vi "Bertta_v09_6.vi"() -> ()   [LabVIEW 2015]
uses:
  x64/Debug/BERTTA.dll
panel:
  out "TIME array":dbl[](array[numeric])
  out "TEMP array":dbl[](array[numeric])
  out "element":bool
  out "Started:":string
  in  "SHUTDOWN":bool
  in  "MASTER CONTROL":bool
  in  "Tab Control":T1(tab)
  in  "Read Seq":bool
  in  "Save Seq":bool
  in  "Configuration file":path=path "C:/Users/shresplab/Desktop/BerttaConfiguration.lvm" caption="Filename"
  in  "OK Button 2":bool
  out "Boolean":bool
  in  "User (initials)":string
  in  "Project name":string
  in  "Description":string
  out "Output file":string
  out "PUMP 3":bool
  out "Target amount":dbl
  out "Scale weight":dbl
  out "Amount now":dbl
  out "Flow rate":dbl
  out "Time to target":dbl format="%<%H:%M:%S>t"
  out "Current step":dbl
  out "Target amount":dbl
  out "Amount now":dbl
  out "Amount now":dbl
  out "Target amount":dbl
  out "Current step":dbl
  out "Time to target":dbl format="%<%H:%M:%S>t"
  out "Flow rate":dbl
  out "Amount now":dbl
  out "Scale weight":dbl
  out "Target amount":dbl
  out "PUMP 2":bool
  out "Sensor OK 6":bool
  out "Sensor OK 5":bool
  out "Sensor OK 4":bool
  out "Sensor OK 3":bool
  in  "OK Button":bool
  in  "Add comment":string
  out "PUMP 1":bool
  out "Target amount":dbl
  out "Scale weight":dbl
  out "Amount now":dbl
  out "Flow rate":dbl
  out "Time to target":dbl format="%<%H:%M:%S>t"
  out "Current step":dbl
  out "Target amount":dbl
  out "Amount now":dbl
  out "Tr":dbl
  out "Tj in":dbl
  out "Tj out":dbl
  out "T set":dbl
  out "Current step":i32
  out "RPM":dbl
  out "Torque 2":dbl
  out "Waveform Chart 5":dynamicdata(graph)
  out "Waveform Chart 6":dynamicdata(graph)
  out "Waveform Chart 7":dynamicdata(graph)
  in  "Tab Control 2":T2(tab)
  out "Waveform Chart 3":dynamicdata(graph)
  out "Waveform Chart 8":dynamicdata(graph)
  out "Waveform Chart 11":dynamicdata(graph)
  out "Waveform Chart 13":dynamicdata(graph)
  out "Waveform Chart 9":dynamicdata(graph)
  out "Table":string[][](table)=[["14.8.2017 18.06.59", "0,000000", "417,670000", "-0,150000", "1,000000", "22,220000", "23,366837", "23,574959", "23,985852", "23,690000", "240,000000", "4,000000", "0,000000", "397,000000", "-397,000000", "1,000000"], ["14.8.2017 18.07.06", "0,000000", "417,640000", "-0,120000", "1,000000", "22,220000", "23,763115", "23,906257", "23,985694", "23,680000", "240,000000", "4,000000", "0,000000", "397,000000", "-397,000000", "1,000000"], ["14.8.2017 18.07.13", "0,000000", "417,640000", "-0,120000", "1,000000", "22,220000", "23,965922", "24,013440", "23,984906", "23,670000", "240,000000", "4,100000", "3,000000", "397,000000", "-397,000000", "1,000000"], ["14.8.2017 18.07.21", "0,000000", "417,640000", "-0,120000", "1,000000", "22,220000", "23,943860", "23,900110", "23,987113", "23,670000", "240,000000", "4,000000", "0,000000", "397,000000", "-397,000000", "1,000000"], ["14.8.2017 18.07.28", "0,000000", "417,640000", "-0,120000", "1,000000", "22,220000", "23,736328", "23,600018", "23,989004", "23,660000", "240,000000", "4,000000", "0,000000", "397,000000", "-397,000000", "1,000000"], ["14.8.2017 18.07.36", "0,000000", "417,640000", "-0,120000", "1,000000", "22,220000", "23,480910", "23,324538", "23,991053", "23,660000", "240,000000", "4,000000", "0,000000", "397,000000", "-397,000000", "1,000000"], ["14.8.2017 18.07.43", "0,000000", "417,640000", "-0,120000", "2,000000", "22,220000", "23,195579", "23,008270", "23,999093", "23,650000", "240,000000", "4,000000", "0,000000", "397,000000", "-397,000000", "1,000000"], ["14.8.2017 18.07.51", "0,000000", "417,650000", "-417,650000", "1,000000", "22,220000", "22,862541", "22,649021", "24,003979", "23,650000", "240,000000", "4,000000", "0,000000", "397,000000", "-397,000000", "2,000000"], ["14.8.2017 18.07.58", "0,000000", "417,640000", "0,010000", "1,000000", "22,220000", "22,541353", "22,354878", "24,005398", "23,650000", "240,000000", "4,000000", "0,000000", "397,000000", "-397,000000", "1,000000"], ["14.8.2017 18.08.06", "0,000000", "417,640000", "0,010000", "1,000000", "22,220000", "22,347931", "22,253738", "24,007605", "23,640000", "240,000000", "4,100000", "0,000000", "397,000000", "-397,000000", "1,000000"], ["14.8.2017 18.08.13", "0,000000", "417,640000", "0,010000", "1,000000", "22,220000", "22,329030", "22,302102", "24,006028", "23,640000", "240,000000", "4,000000", "0,000000", "395,820000", "-395,820000", "1,000000"], ["14.8.2017 18.08.20", "0,000000", "417,640000", "0,010000", "1,000000", "22,220000", "22,466849", "22,511320", "24,002403", "23,630000", "240,000000", "4,000000", "0,000000", "395,830000", "-0,010000", "1,000000"], ["14.8.2017 18.08.28", "0,000000", "417,640000", "0,010000", "1,000000", "22,220000", "22,707062", "22,835101", "24,000984", "23,620000", "240,000000", "4,000000", "0,000000", "395,830000", "-0,010000", "1,000000"], ["14.8.2017 18.08.35", "0,000000", "417,640000", "0,010000", "1,000000", "22,220000", "23,054104", "23,232979", "24,001299", "23,600000", "240,000000", "4,000000", "0,000000", "395,830000", "-0,010000", "1,000000"], ["14.8.2017 18.08.43", "0,000000", "417,640000", "0,010000", "1,000000", "22,220000", "23,412371", "23,522793", "24,002560", "23,590000", "240,000000", "4,000000", "0,000000", "395,820000", "0,000000", "1,000000"], ["14.8.2017 18.08.51", "0,000000", "417,640000", "0,010000", "1,000000", "22,220000", "23,596247", "23,656125", "24,003821", "23,580000", "240,000000", "4,000000", "0,000000", "395,820000", "0,000000", "1,000000"]]
  in  "Reset":bool
  in  "Numeric 4":dbl=20.0
  in  "Numeric 3":dbl=30.0
  in  "Numeric 2":dbl=40.0
  in  "Numeric 1":dbl=30.0
  in  "Numeric":dbl=20.0
  out "Boolean 12":bool
  out "Boolean 7":bool
  out "Boolean 6":bool
  out "Boolean 5":bool
  out "Boolean 4":bool
  out "Boolean 19":bool
  in  "Numeric 5":dbl=5.0
  in  "Numeric 6":dbl=5.0
  in  "Numeric 7":dbl=5.0
  in  "Numeric 8":dbl=5.0
  in  "T ext / T ext 2":enum32{"External 1", "External 2"}(radio)
  out "Sensor OK":bool
  in  "T fail":dbl=20.0
  in  "?":bool
  in  "T manual setpoint":dbl=20.0
  in  "Lauda port":dbl=9.0
  in  "Manual select":enum32{"Tr", "Tj"}(radio)
  in  "PAUSE":bool
  out "Waveform Chart":dynamicdata(graph)
  out "T external 2":dbl
  out "result":bool
  out "Led11 5":bool
  in  "Port":i32=10
  in  "Radio Buttons 4":enum32{"Reglo Digital", "Reglo Analog", "PAM"}(radio)
  out "Speed":dbl
  out "mA":dbl format="%#_2g"
  in  "Port":i32=16
  out "RPM":dbl format="%_4f"
  out "Led10 3":bool
  out "Led9 3":bool
  out "Led8 3":bool
  out "Led7 3":bool
  out "Led6 3":bool
  out "Led5 3":bool
  out "Led4 3":bool
  out "Led3 3":bool
  out "Led2 3":bool
  out "Led1 3":bool
  in  "PumpSeq 4":dbl[][](array[numeric])=[[1.0, 1.0, 7.0], [2.0, 1.0, 2.0], [3.0, 1.0, 100.0], [0.0, 0.0, 0.0], [0.0, 0.0, 0.0], [0.0, 0.0, 0.0], [0.0, 0.0, 0.0], [0.0, 0.0, 0.0], [0.0, 0.0, 0.0], [0.0, 0.0, 0.0], [0.0, 1.0, 0.0]]
  in  "?":bool
  out "Flow rate (g/min)":dbl
  out "Scale reading":dbl
  out "Step amount now":dbl
  in  "Grams / min":dbl
  out "Waveform Chart 14":dynamicdata(graph)
  in  "?":bool
  out "Total amount now":dbl
  out "Total time 4":dbl
  out "Total amount target 4":dbl
  out "Led11 4":bool
  in  "Reset 5":bool
  out "elapsed / step":i32
  out "Time to target":dbl format="%<%H:%M:%S>t"
  out "Led11":bool
  in  "Port":i32=11
  in  "Radio Buttons 2":enum32{"Reglo Digital", "Reglo Analog", "PAM"}(radio)
  out "Speed":dbl
  out "mA":dbl format="%#_2g"
  in  "Port":i32=15
  out "RPM":dbl format="%_4f"
  out "Led10":bool
  out "Led9":bool
  out "Led8":bool
  out "Led7":bool
  out "Led6":bool
  out "Led5":bool
  out "Led4":bool
  out "Led3":bool
  out "Led2":bool
  out "Led1":bool
  in  "PumpSeq 2":dbl[][](array[numeric])=[[1.0, 1.0, 7.0], [2.0, 1.0, 2.0], [3.0, 1.0, 100.0], [0.0, 0.0, 0.0], [0.0, 0.0, 0.0], [0.0, 0.0, 0.0], [0.0, 0.0, 0.0], [0.0, 0.0, 0.0], [0.0, 0.0, 0.0], [0.0, 0.0, 0.0], [0.0, 1.0, 0.0]]
  in  "?":bool
  out "Flow rate (g/min)":dbl
  out "Scale reading":dbl
  out "Step amount now":dbl
  in  "Grams / min":dbl
  out "Waveform Chart 10":dynamicdata(graph)
  in  "?":bool
  out "Total amount now":dbl
  out "Total time 2":dbl
  out "Total amount target 2":dbl
  out "Led11":bool
  in  "Reset 3":bool
  out "elapsed / step":i32
  out "Time to target":dbl format="%<%H:%M:%S>t"
  out "Led11 3":bool
  in  "Port":i32=12
  in  "Radio Buttons 3":enum32{"Reglo Digital", "Reglo Analog", "PAM"}(radio)
  out "Speed":dbl
  out "mA":dbl format="%#_2g"
  in  "Port":i32=14
  out "RPM":dbl format="%_4f"
  out "Led10 2":bool
  out "Led9 2":bool
  out "Led8 2":bool
  out "Led7 2":bool
  out "Led6 2":bool
  out "Led5 2":bool
  out "Led4 2":bool
  out "Led3 2":bool
  out "Led2 2":bool
  out "Led1 2":bool
  in  "PumpSeq 3":dbl[][](array[numeric])=[[1.0, 1.0, 7.0], [2.0, 1.0, 2.0], [3.0, 1.0, 100.0], [0.0, 0.0, 0.0], [0.0, 0.0, 0.0], [0.0, 0.0, 0.0], [0.0, 0.0, 0.0], [0.0, 0.0, 0.0], [0.0, 0.0, 0.0], [0.0, 0.0, 0.0], [0.0, 1.0, 0.0]]
  in  "?":bool
  out "Flow rate (g/min)":dbl
  out "Scale reading":dbl
  out "Step amount now":dbl
  in  "Grams / min":dbl
  out "Waveform Chart 12":dynamicdata(graph)
  in  "?":bool
  out "Total amount now":dbl
  out "Total time 3":dbl
  out "Total amount target 3":dbl
  out "Led11 2":bool
  in  "Reset 4":bool
  out "elapsed / step":i32
  out "Time to target":dbl format="%<%H:%M:%S>t"
  in  "Bypass select 2":enum32{"Remote", "Manual"}(radio)=enum."Manual"
  in  "Port":dbl=13.0
  out "RPM":dbl
  out "Torque":dbl
  in  "Set RPM":dbl(slide) scale=0.0..2000.0
  out "Waveform Chart 4":dynamicdata(graph)
  out "DAQ 9217 (PT100)":errorcluster
  # "Temperature sensor:"
  # "Manual control:"
  # "PUMP & SCALE 1"
  # "STEP"
  # "TOTAL"
  # "PUMP & SCALE 2"
  # "STEP"
  # "TOTAL"
  # "PUMP & SCALE 3"
  # "STEP"
  # "TOTAL"
  # "Manual control"
  # "Secondary temperature sensor"
  # "Device communication"
  # "Temp"
  # "Time"
  # "Grams    /   min"
  # "End of sequence"
  # "Manual control"
  # "Device communication"
  # "Pump configuration"
  # "Scale configuration"
  # "SCALE 1"
  # "Grams    /   min"
  # "End of sequence"
  # "Manual control"
  # "Device communication"
  # "Pump configuration"
  # "Scale configuration"
  # "SCALE 2"
  # "Grams    /   min"
  # "End of sequence"
  # "Manual control"
  # "Device communication"
  # "Pump configuration"
  # "Scale configuration"
  # "SCALE 3"
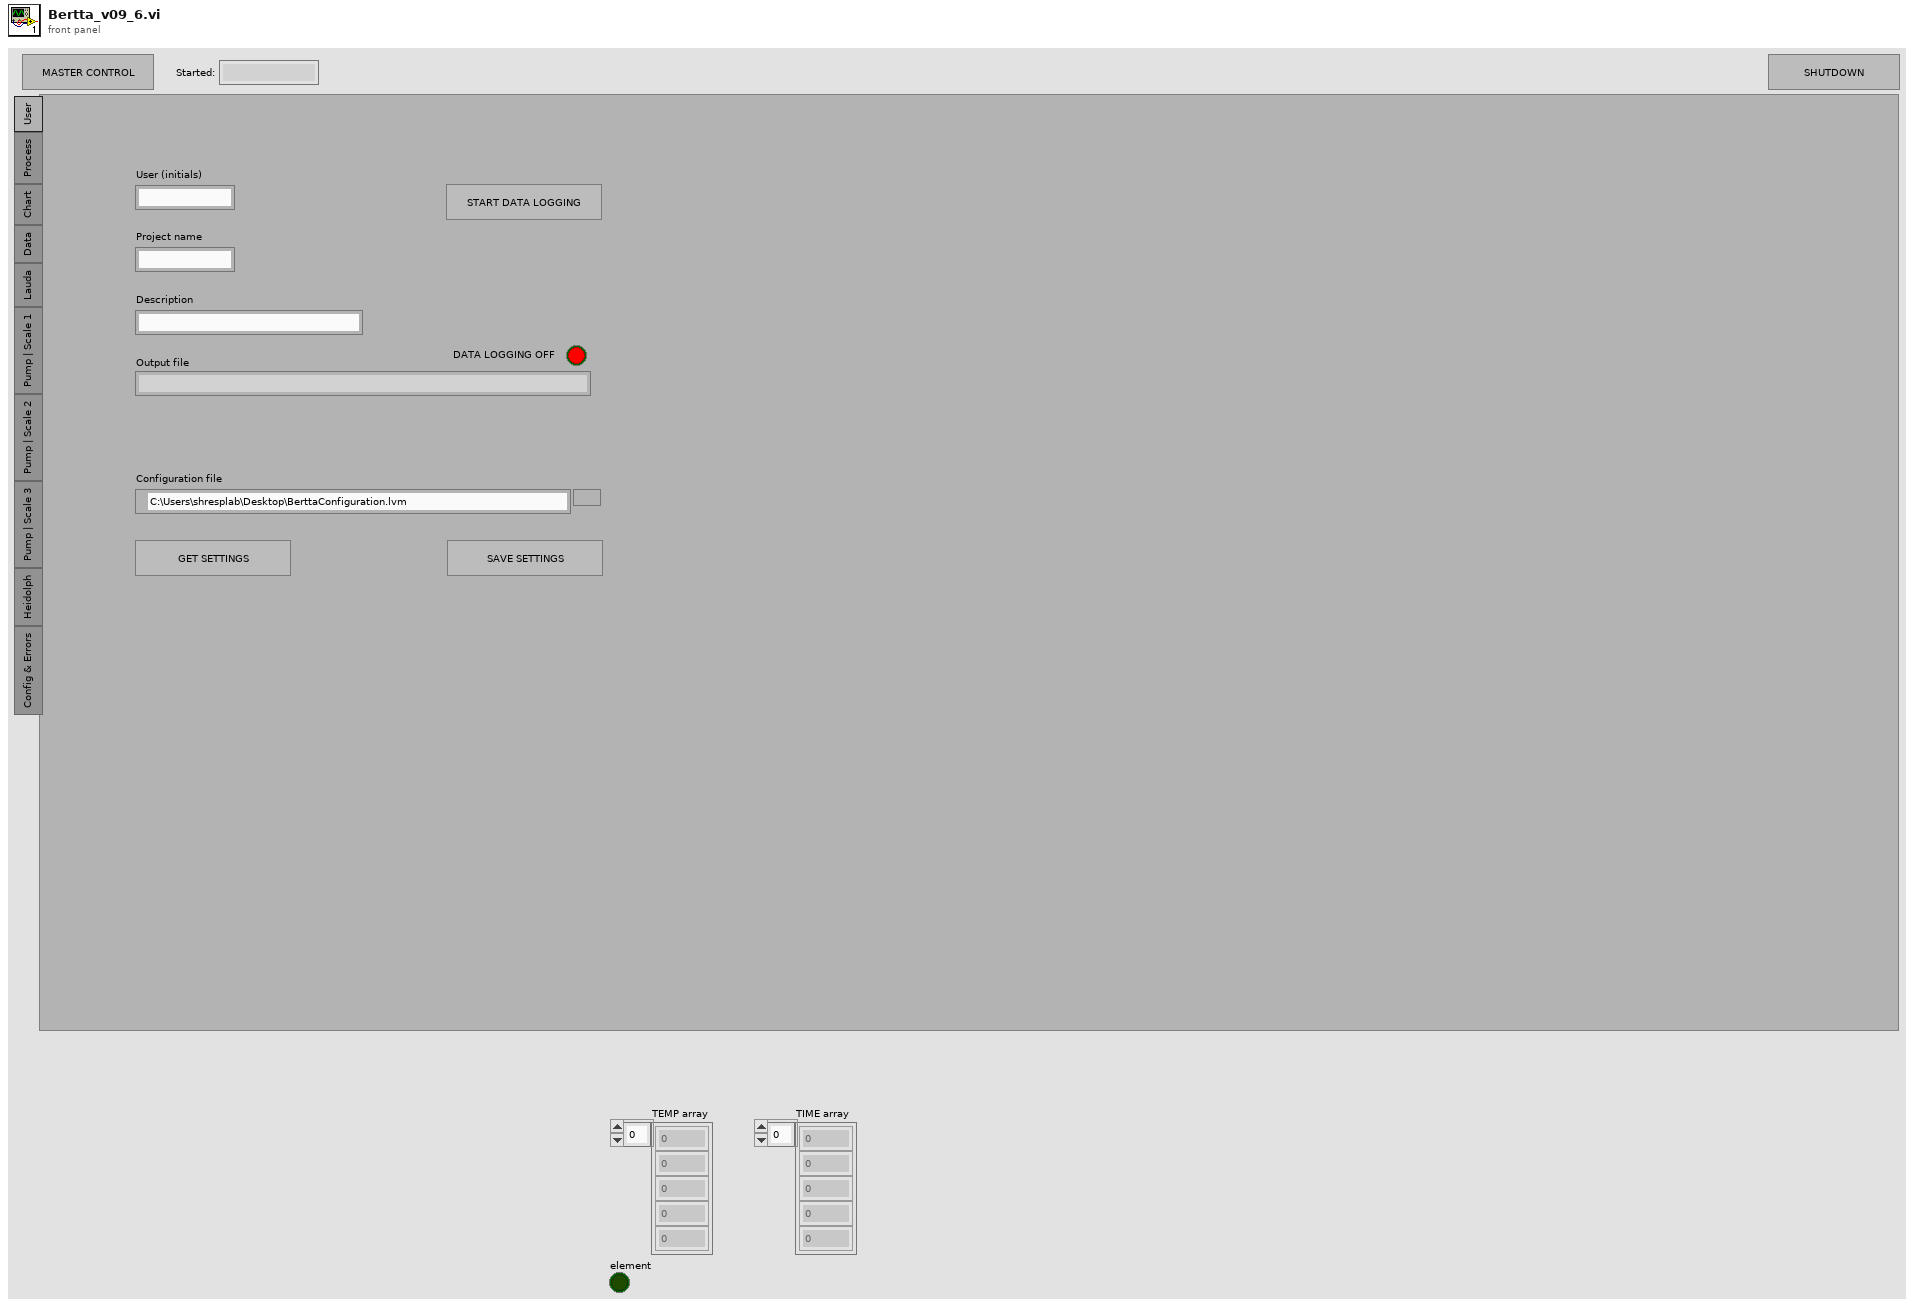
[diagram p1: front panel]
types:
  T1 = enum32{"User", "Process", "Chart", "Data", "Lauda", "Pump | Scale 1", "Pump | Scale 2", "Pump | Scale 3", "Heidolph", "Config & Errors"}
  T2 = enum32{"Temperatures", "Scale / Pump 1", "Scale / Pump 2", "Scale / Pump 3", "RPM / torque"}
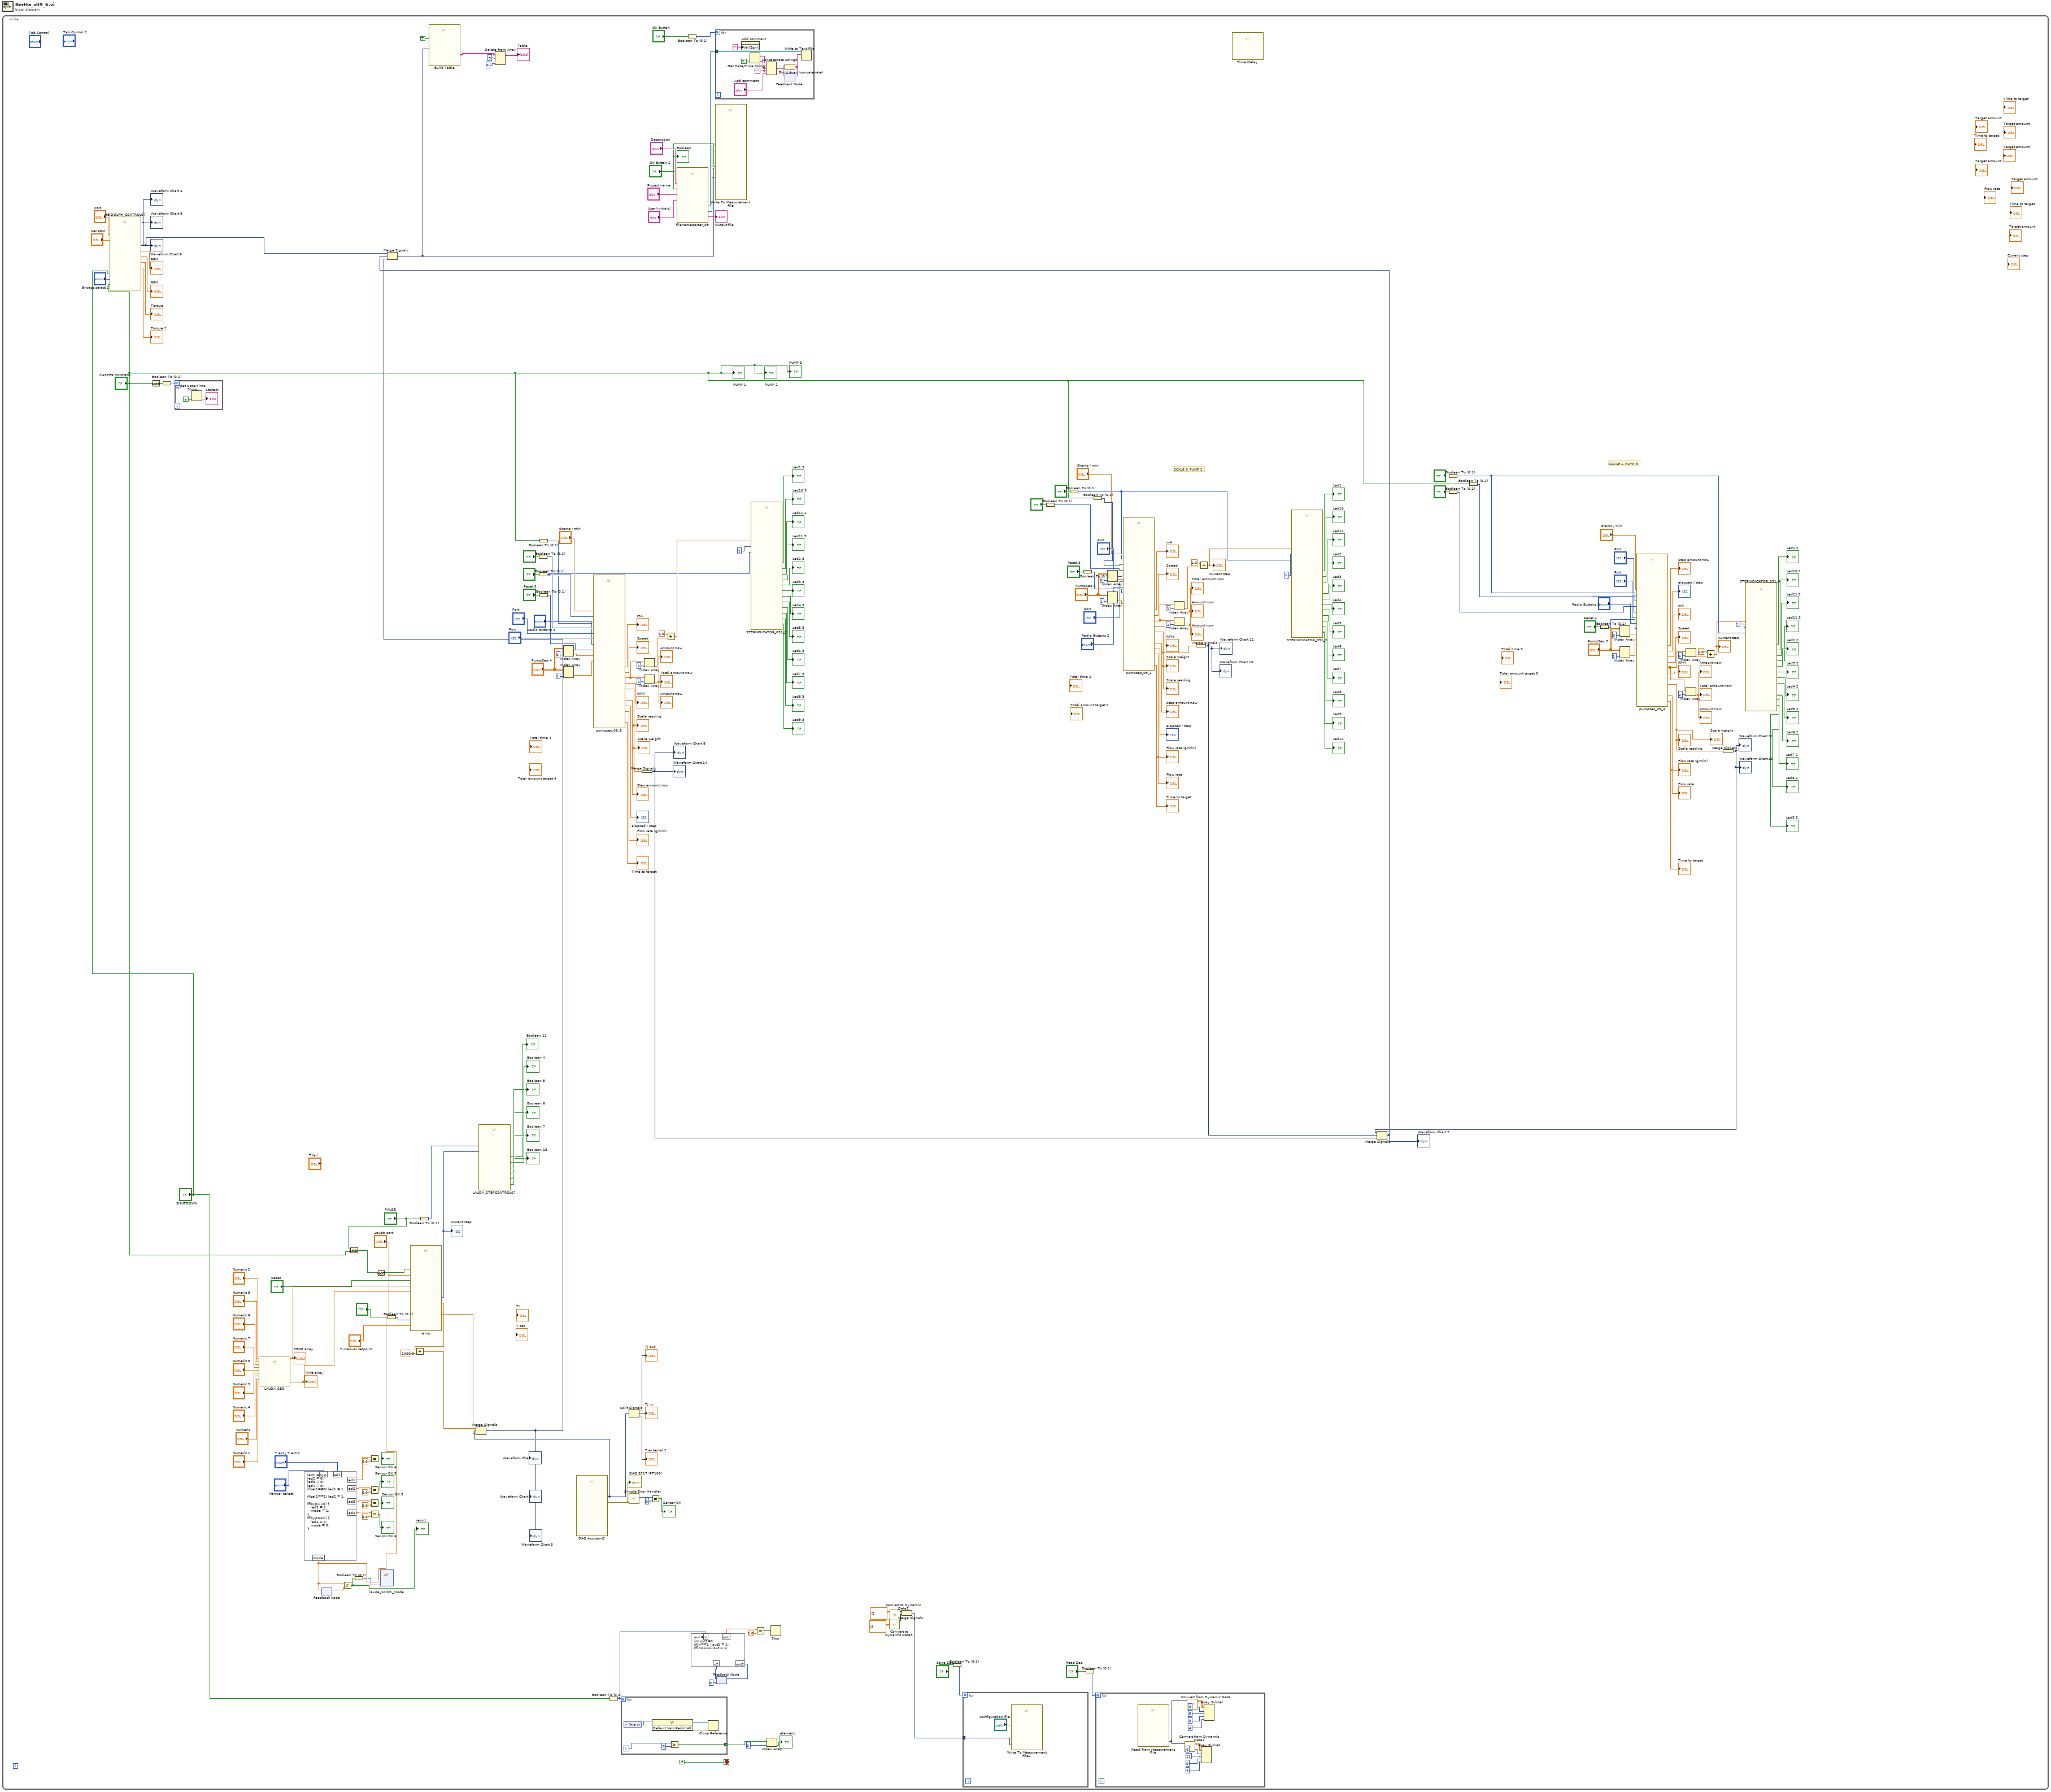
[diagram p0: block diagram]
diagram:
  n1 = while {
    stop <- FALSE stop-if-true
    # "SCALE & PUMP 3"
    # "SCALE & PUMP 2"
    n2 = call "HEIDOLPH_CONTROL07.vi"("master"="MASTER CONTROL", "shutdown"="SHUTDOWN", "Bypass select"="Bypass select 2", "Set RPM"="Set RPM", "Device port"="Port") -> ("Dynamic Data"=w235:dynamicdata, "RPM"=→"RPM":dbl, "RPM 2"=→"RPM":dbl, "Torque"=→"Torque":dbl, "Torque 2"=→"Torque 2":dbl)  [unwired: 2 in]
    "Waveform Chart 4" <- w235
    "Waveform Chart 6" <- w235
    "Waveform Chart 9" <- w235
    n3 = Not(x="MASTER CONTROL") -> (.not. x?=w220:bool)
    n4 = Boolean To (0,1)(Boolean=w220) -> (0, 1=w221:i16)
    n5 = for {
      N: w221 -> [_]
      n6 = Get Date/Time String(want seconds? (F)=TRUE) -> (time string=→"Started:":string)  [unwired: 2 in, 1 out]
    }
    n7 = call "LAUDA_SEQ.vi"("Numeric 2"="Numeric 2", "Numeric 1"="Numeric 1", "Numeric"="Numeric", "Numeric 5"="Numeric 5", "Numeric 6"="Numeric 6", "Numeric 7"="Numeric 7", "Numeric 8"="Numeric 8", "Numeric 3"="Numeric 3", "Numeric 4"="Numeric 4") -> ("output array"=w113:dbl[], "output array 2"=w112:dbl[])  [unwired: 5 in]
    "TEMP array" <- w113
    "TIME array" <- w112
    n8 = formula code="led1 = 0;\nled2 = 0;\nled3 = 0;\nled4 = 0;\nif(sel1==0) led1 = 1;\n\nif(sel1==1) led2 = 1;\n\nif(byp==0) {\n   led3 = 1;\n   mode = 1;\n}\nif(byp==1) {\n   led4 = 1;\n   mode = 0;\n}"("sel1"="T ext / T ext 2", "byp"="Manual select") -> ("led1"=w190:dbl, "led2"=w188:dbl, "led3"=w183:dbl, "led4"=w182:dbl, "mode"=w106:dbl)
    n9 = feedback-in #1(w106) -> ()
    n10 = feedback #1() -> (w105:dbl)  [unwired: 1 in]
    n11 = Not Equal?(x=w106, y=w105) -> (x != y?=w103:bool)
    "result" <- w103
    n12 = And(x="PAUSE", y="MASTER CONTROL") -> (x .and. y?=w125:bool)
    n13 = Boolean To (0,1)(Boolean=w103) -> (0, 1=w104:i16)
    n14 = Equal?(x=w190, y=0.0) -> (x = y?=→"Sensor OK 4":bool)
    n15 = Equal?(x=w188, y=0.0) -> (x = y?=→"Sensor OK 3":bool)
    n16 = Equal?(x=w183, y=0.0) -> (x = y?=→"Sensor OK 5":bool)
    n17 = Equal?(x=w182, y=0.0) -> (x = y?=→"Sensor OK 6":bool)
    n18 = Not(x=w125) -> (.not. x?=w124:bool)
    n19 = dll-call lib="C:/Users/shresplab/OneDrive - Kemira Oyj/Documents/Visual Studio 2017/Projects/Bertta/BERTTA/x64/Debug/BERTTA.dll" fn="lauda_switch_mode"("port"="Lauda port", "mode"=w106, "enable"=w104) -> ()  [unwired: 7 in, 2 out]
    n20 = Boolean To (0,1)(Boolean="?") -> (0, 1=w109:i16)
    n21 = call "ramp.vi"("TimeParams"=w112, "Seq"=w113, "T_man"="T manual setpoint", "manual"=w109, "port"="Lauda port", "reset"="Reset", "pause"=w124) -> ("T control"=w128:dbl, "STEP"=w130:i32, "T ext"=w111:dbl)  [unwired: 1 in, 1 out]
    "Current step" <- w130
    n22 = Divide(x=w128, y=1000.0) -> (x/y=w127:dbl)
    n23 = Boolean To (0,1)(Boolean="PAUSE") -> (0, 1=w177:i16)
    n24 = call "LAUDA_STEPCONTROL07.vi"("step"=w130, "pause"=w177) -> ("Boolean 13"=→"Boolean 19":bool, "Boolean 6"=→"Boolean 6":bool, "Boolean 5"=→"Boolean 5":bool, "Boolean 4"=→"Boolean 4":bool, "Boolean 7"=→"Boolean 7":bool, "Boolean 12"=→"Boolean 12":bool)  [unwired: 4 in]
    n25 = Boolean To (0,1)(Boolean="?") -> (0, 1=w13:i16)
    n26 = Boolean To (0,1)(Boolean="?") -> (0, 1=w23:i16)
    n27 = Boolean To (0,1)(Boolean="MASTER CONTROL") -> (0, 1=w2:i16)
    n28 = Boolean To (0,1)(Boolean="Reset 5") -> (0, 1=w22:i16)
    n29 = Index Array(array="PumpSeq 4", index (col)=0) -> (element=w28:dbl[])  [unwired: 1 in]
    n30 = Index Array(array="PumpSeq 4", index (col)=1) -> (element=w50:dbl[])  [unwired: 1 in]
    n31 = call "DAQ Assistant2"() -> ("data"=w137:dynamicdata, "error out"=w230:errorcluster)  [unwired: 17 in, 1 out]
    "DAQ 9217 (PT100)" <- w230
    n32 = Merge Signals(w127, w137, w111) -> (w136:dynamicdata)
    "Waveform Chart 3" <- w136
    "Waveform Chart" <- w136
    "Waveform Chart 5" <- w136
    n33 = call "pumpsec_09_5.vi"("reset"=w22, "master"=w2, "manual"=w13, "pause"=w23, "Port"="Port", "pump_type"="Radio Buttons 4", "port, Reglo D"="Port", "Target"=w28, "fr_manual"="Grams / min", "Time"=w50) -> ("time_to_target"=→"Time to target":dbl, "step_fr"=→"Flow rate (g/min)":dbl, "amount_step"=→"Step amount now":dbl, "Reglo D"=→"RPM":dbl, "Scale"=w5:dbl, "mA"=→"mA":dbl, "elapsed_step"=→"elapsed / step":dbl, "params"=w47:dbl[], "PAM"=→"Speed":dbl)  [unwired: 7 in, 2 out]
    "Scale weight" <- w5
    "Scale reading" <- w5
    n34 = Boolean To (0,1)(Boolean="SHUTDOWN") -> (0, 1=w195:i16)
    n35 = for {
      N: w195 -> [_]
      tunnel: [w265] -> w219 mode=indexing
      i -> [w267]
      n36 = control-ref of="This VI"() -> (w270:refnum<vi>)
      n37 = invoke class="VI" method="Default Vals.Reinit All"(reference=w270) -> (reference out=w268:refnum<vi>, error out=w269:errorcluster)  [unwired: 2 in, 1 out]
      n38 = Greater?(x=w267, y=0) -> (0:w265:bool)
      n39 = Close Reference(reference=w268, error in (no error)=w269) -> ()  [unwired: 1 out]
    }
    n40 = Split Signals(w137) -> (→"Tj out":dynamicdata, →"Tj in":dynamicdata, →"T external 2":dynamicdata)  [unwired: 3 in]
    n41 = call <vilib>:"Simple Error Handler.vi"("error in (no error)"=w230) -> ("code out"=w229:i32)  [unwired: 4 in, 4 out]
    n42 = Merge Signals(w5) -> (w3:dynamicdata)
    "Waveform Chart 8" <- w3
    "Waveform Chart 14" <- w3
    n43 = Index Array(array=w47, index=1) -> (element=w44:dbl)
    n44 = Index Array(array=w47, index=2) -> (element=→"Amount now" →"Amount now" →"Total amount now":dbl)
    n45 = Not Equal?(x=w229, y=0) -> (x != y?=→"Sensor OK":bool)
    n46 = Add(x=1.0, y=w44) -> (x+y=w43:dbl)
    n47 = call "filenameparser_09.vi"("Description"="Description", "Project name"="Project name", "User (initials)"="User (initials)", "OK Button in"="OK Button 2") -> ("Output file"=→"Output file":string, "appended path 2"=w202:path, "appended path"=w201:path)  [unwired: 5 in]
    n48 = Boolean To (0,1)(Boolean="OK Button") -> (0, 1=w200:i16)
    n49 = for {
      N: w200 -> [_]
      tunnel: w201 -> [w244]
      w248 = " " ("string")
      n50 = property on="Add comment" class="Str"("Val(Sgnl)"="" ("Value (Signaling)")) -> ()  [unwired: 2 in, 2 out]
      n51 = Get Date/Time String(want seconds? (F)=TRUE) -> (date string=w251:string, time string=w249:string)  [unwired: 2 in]
      n52 = Concatenate Strings(w251, w248, w249, w248, "Add comment") -> (w247:string)
      n53 = feedback #2() -> (w246:string[])  [unwired: 1 in]
      n54 = Build Array (concatenate)(w246, w247) -> (w245:string[])
      n55 = feedback-in #2(w245) -> ()
      n56 = Write to Text File(file (use dialog)=w244, text=w245) -> ()  [unwired: 2 in, 3 out]
    }
    n57 = feedback #3(0) -> (w193:i32)
    n58 = formula code="out = 0;\nint out2=0;\nif(in==1 ) out2 = 1;\nif(in2==1) out = 1;"("in"=w195, "in2"=w193) -> ("out"=w197:dbl, "out2"=w194:i32)
    n59 = feedback-in #3(w194) -> ()
    n60 = call "STEPINDICATOR_091_2.vi"("current step"=w43, "enable"=i16 1, "manual"=w13) -> ("Led 8"=→"Led8 3":bool, "Led 10"=→"Led10 3":bool, "Led 11"=→"Led11 4":bool, "Led 7"=→"Led7 3":bool, "Led 1"=→"Led1 3":bool, "Led 6"=→"Led6 3":bool, "Led 2"=→"Led2 3":bool, "Led 12"=→"Led11 5":bool, "Led 5"=→"Led5 3":bool, "Led 4"=→"Led4 3":bool, "Led 3"=→"Led3 3":bool, "Led 9"=→"Led9 3":bool)  [unwired: 1 in]
    n61 = Equal?(x=w197, y=1.0) -> (x = y?=w196:bool)
    n62 = Index Array(array=w219, index=0) -> (element=→"element":bool)
    n63 = Stop(stop? (T)=w196) -> ()
    n64 = call "Convert to Dynamic Data3"("2D Array"=dbl[][] []) -> ("Dynamic Data Type"=w179:dynamicdata)  [unwired: 3 in]
    n65 = call "Convert to Dynamic Data2"("2D Array"=dbl[][] []) -> ("Dynamic Data Type"=w217:dynamicdata)  [unwired: 3 in]
    n66 = Merge Signals(w217, w179) -> (w216:dynamicdata)
    n67 = Boolean To (0,1)(Boolean="Save Seq") -> (0, 1=w215:i16)
    n68 = for {
      N: w215 -> [_]
      tunnel: w216 -> [w264]
      n69 = call "Write To Measurement File2"("Signals"=w264, "Filename"="Configuration file") -> ()  [unwired: 15 in, 3 out]
    }
    n70 = Boolean To (0,1)(Boolean="?") -> (0, 1=w166:i16)
    n71 = Boolean To (0,1)(Boolean="?") -> (0, 1=w94:i16)
    n72 = Boolean To (0,1)(Boolean="Reset 3") -> (0, 1=w163:i16)
    n73 = Boolean To (0,1)(Boolean="Read Seq") -> (0, 1=w212:i16)
    n74 = Boolean To (0,1)(Boolean="MASTER CONTROL") -> (0, 1=w157:i16)
    n75 = for {
      N: w212 -> [_]
      n76 = call "Read From Measurement File"() -> ("Signals"=w253:dynamicdata)  [unwired: 6 in, 5 out]
      n77 = call "Convert from Dynamic Data2"("Dynamic Data Type"=w253) -> ("Array"=w252:dbl[][])  [unwired: 3 in]
      n78 = call "Convert from Dynamic Data"("Dynamic Data Type"=w253) -> ("Array"=w260:dbl[][])  [unwired: 3 in]
      n79 = Array Subset(array=w252, index (row)=6 ("index"), length (row)=11 ("length"), index (col)=0 ("index"), length (col)=4 ("length")) -> ()  [unwired: 1 out]
      n80 = Array Subset(array=w260, index (row)=0 ("index"), length (row)=6 ("length"), index (col)=0 ("index"), length (col)=4 ("length")) -> ()  [unwired: 1 out]
    }
    n81 = Index Array(array="PumpSeq 2", index (col)=0 ("disabled index (col)")) -> (element=w169:dbl[])  [unwired: 1 in]
    n82 = Index Array(array="PumpSeq 2", index (col)=1 ("disabled index (col)")) -> (element=w168:dbl[])  [unwired: 1 in]
    n83 = call "pumpsec_09_2.vi"("reset"=w163, "master"=w157, "manual"=w94, "pause"=w166, "Port"="Port", "pump_type"="Radio Buttons 2", "port, Reglo D"="Port", "Target"=w169, "fr_manual"="Grams / min", "Time"=w168) -> ("time_to_target"=→"Time to target":dbl, "step_fr"=→"Flow rate" →"Flow rate (g/min)":dbl, "amount_step"=→"Step amount now":dbl, "Reglo D"=→"RPM":dbl, "Scale"=w101:dbl, "mA"=→"mA":dbl, "elapsed_step"=→"elapsed / step":dbl, "params"=w158:dbl[], "PAM"=→"Speed":dbl)  [unwired: 7 in, 2 out]
    "Scale weight" <- w101
    "Scale reading" <- w101
    n84 = Index Array(array=w158, index=1) -> (element=w161:dbl)
    n85 = Index Array(array=w158, index=2) -> (element=→"Amount now" →"Amount now" →"Total amount now":dbl)
    n86 = Merge Signals(w101) -> (w6:dynamicdata)
    "Waveform Chart 11" <- w6
    "Waveform Chart 10" <- w6
    n87 = Add(x=1.0, y=w161) -> (x+y=w151:dbl)
    "Current step" <- w151
    n88 = call "Time Delay"() -> ()  [unwired: 11 in, 1 out]
    n89 = call "STEPINDICATOR_091_2.vi"("current step"=w151, "enable"=i16 1, "manual"=w94) -> ("Led 8"=→"Led8":bool, "Led 10"=→"Led10":bool, "Led 11"=→"Led11":bool, "Led 7"=→"Led7":bool, "Led 1"=→"Led1":bool, "Led 6"=→"Led6":bool, "Led 2"=→"Led2":bool, "Led 12"=→"Led11":bool, "Led 5"=→"Led5":bool, "Led 4"=→"Led4":bool, "Led 3"=→"Led3":bool, "Led 9"=→"Led9":bool)  [unwired: 1 in]
    n90 = Boolean To (0,1)(Boolean="?") -> (0, 1=w88:i16)
    n91 = Boolean To (0,1)(Boolean="?") -> (0, 1=w87:i16)
    n92 = Boolean To (0,1)(Boolean="MASTER CONTROL") -> (0, 1=w89:i16)
    n93 = Boolean To (0,1)(Boolean="Reset 4") -> (0, 1=w67:i16)
    n94 = Index Array(array="PumpSeq 3", index (col)=0 ("disabled index (col)")) -> (element=w71:dbl[])  [unwired: 1 in]
    n95 = Index Array(array="PumpSeq 3", index (col)=1 ("disabled index (col)")) -> (element=w70:dbl[])  [unwired: 1 in]
    n96 = call "pumpsec_09_4.vi"("reset"=w67, "master"=w89, "manual"=w88, "pause"=w87, "Port"="Port", "pump_type"="Radio Buttons 3", "port, Reglo D"="Port", "Target"=w71, "fr_manual"="Grams / min", "Time"=w70) -> ("time_to_target"=→"Time to target":dbl, "step_fr"=→"Flow rate" →"Flow rate (g/min)":dbl, "amount_step"=→"Step amount now":dbl, "Reglo D"=→"RPM":dbl, "Scale"=w10:dbl, "mA"=→"mA":dbl, "elapsed_step"=→"elapsed / step":dbl, "params"=w53:dbl[], "PAM"=→"Speed":dbl)  [unwired: 7 in, 2 out]
    "Scale weight" <- w10
    "Scale reading" <- w10
    n97 = Index Array(array=w53, index=1) -> (element=w54:dbl)
    n98 = Index Array(array=w53, index=2) -> (element=→"Amount now" →"Amount now" →"Total amount now":dbl)
    n99 = Add(x=1.0, y=w54) -> (x+y=w51:dbl)
    "Current step" <- w51
    n100 = Merge Signals(w10) -> (w4:dynamicdata)
    "Waveform Chart 13" <- w4
    "Waveform Chart 12" <- w4
    n101 = Merge Signals(w4, w6, w3) -> (w138:dynamicdata)
    "Waveform Chart 7" <- w138
    n102 = Merge Signals(w235, w138, w136) -> (w207:dynamicdata)
    n103 = call "Build Table"("Include time data"=TRUE, "Signals"=w207) -> ("Table"=w206:string[][])  [unwired: 3 in, 6 out]
    n104 = Delete From Array(array=w206, length=9, index (col)=0 ("index (row)")) -> (array with subset deleted=→"Table":string[][])  [unwired: 1 in, 1 out]
    n105 = call "Write To Measurement File"("Signals"=w207, "Enable"="OK Button 2", "Filename"=w202) -> ()  [unwired: 14 in, 3 out]
    n106 = call "STEPINDICATOR_091_4.vi"("current step"=w51, "enable"=i16 1, "manual"=w88) -> ("Led 8"=→"Led8 2":bool, "Led 10"=→"Led10 2":bool, "Led 11"=→"Led11 2":bool, "Led 7"=→"Led7 2":bool, "Led 1"=→"Led1 2":bool, "Led 6"=→"Led6 2":bool, "Led 2"=→"Led2 2":bool, "Led 12"=→"Led11 3":bool, "Led 5"=→"Led5 2":bool, "Led 4"=→"Led4 2":bool, "Led 3"=→"Led3 2":bool, "Led 9"=→"Led9 2":bool)  [unwired: 1 in]
    "PUMP 1" <- "MASTER CONTROL"
    "Boolean" <- "OK Button 2"
    "PUMP 2" <- "MASTER CONTROL"
    "PUMP 3" <- "MASTER CONTROL"
  }
